vi "Extract name.vi"() -> ()   [LabVIEW 2015]
uses:
  <vilib>/Utility/file.llb/Write Delimited Spreadsheet (string).vi
panel:
  in  "base path":path=path "F:/fh/传输D/2015谷粒实验/提取数据/后期处理数据/1-8综合"
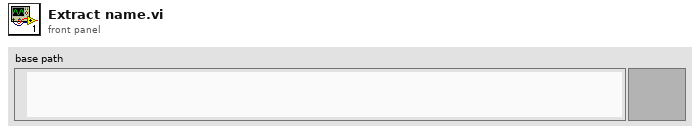
[diagram p1: front panel]
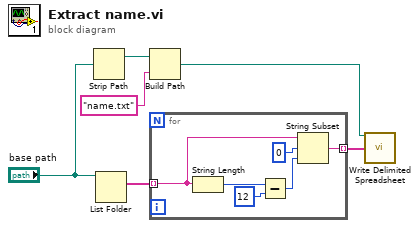
[diagram p0: block diagram]
diagram:
  n1 = Strip Path(path="base path") -> (stripped path=w4:path)  [unwired: 1 out]
  n2 = List Folder(path="base path") -> (filenames=w6:string[])  [unwired: 3 in, 3 out]
  n3 = Build Path(base path=w4, name or relative path="name.txt") -> (appended path=w2:path)
  n4 = for {
    tunnel: w6 -> [w12] mode=indexing
    tunnel: [w7] -> w1 mode=indexing
    n5 = String Length(string=w12) -> (length=w11:i32)
    n6 = Subtract(x=w11, y=12) -> (x-y=w8:i32)
    n7 = String Subset(string=w12, offset (0)=0, length (rest)=w8) -> (substring=w7:string)
  }
  n8 = call-poly <vilib>:"Write Delimited Spreadsheet.vi"("file path (dialog if empty)"=w2, "1D data"=w1) -> ()  [unwired: 12 in, 2 out]
